vi "Get_Folders_Client.vi"(0 "Relative Path":path) -> (1 "Folder Names":string[](array[string]), 2 "error out":errorcluster)   [LabVIEW 2013]
uses:
  Anemometry/Anemometry Sub Vis/Globals/Preference_global.vi
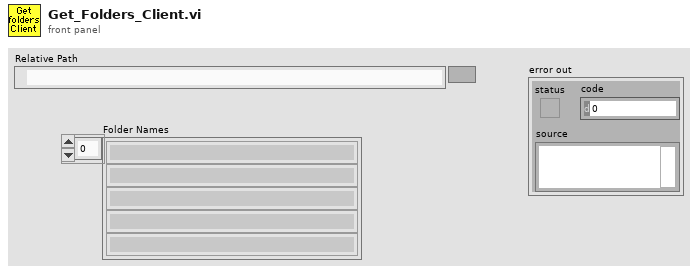
[diagram p1: front panel]
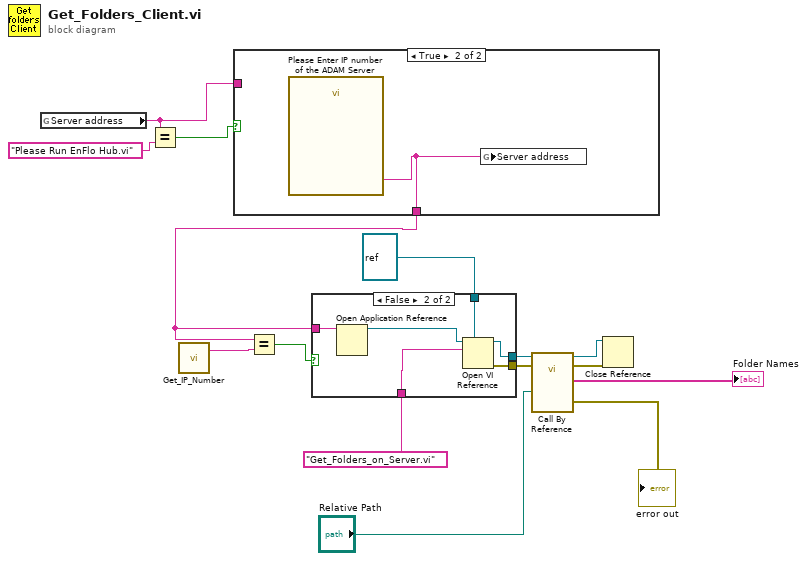
[diagram p0: block diagram]
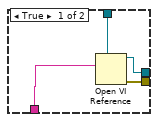
[diagram p3: hidden frame]
diagram:
  n1 = global read "Preference_global.vi" "Server address"() -> (w1:string)
  n2 = Equal?(x=w1, y="Please Run EnFlo Hub.vi" ("Server address")) -> (x = y?=w3:bool)
  n3 = call "Get_IP_Number.vi"() -> ("IP Number"=w9:string)  [unwired: 1 out]
  n4 = case shown="True" w3 {
    tunnel: [w16 w17] -> w2
    tunnel: w1 -> [w16 _]
    frame False {
    }
    frame True {
      n5 = call "Please Enter IP number of the ADAM Server"() -> ("Server IP Number"=w17:string)  [unwired: 17 in, 2 out]
      n6 = global write "Preference_global.vi" "Server address"(w17) -> ()
    }
  }
  n7 = Equal?(x=w2, y=w9) -> (x = y?=w8:bool)
  n8 = case shown="False" w8 {
    tunnel: [w21 w27] -> w10
    tunnel: [w20 w26] -> w11
    tunnel: "Get_Folders_on_Server.vi" -> [w19 w25]
    tunnel: refnum<vi> refnum ("Scout Server") -> [w18 w24]
    tunnel: w2 -> [_ w23]
    frame True {
      n9 = Open VI Reference(type specifier VI Refnum (for type only)=w18, vi path=w19) -> (vi reference=w21:refnum<vi>, error out=w20:errorcluster)  [unwired: 2 in, 2 out]
    }
    frame False {
      n10 = Open Application Reference(11:w23) -> (3:w22:refnum<vi>)  [unwired: 2 in, 2 out]
      n11 = Open VI Reference(type specifier VI Refnum (for type only)=w24, application reference (local)=w22, vi path=w25) -> (vi reference=w27:refnum<vi>, error out=w26:errorcluster)  [unwired: 1 in, 2 out]
    }
  }
  n12 = call-by-ref "?"(reference=w10, error in=w11, "Relative Path"="Relative Path") -> (reference out=w12:refnum<vi>, error out=w15:errorcluster, "Folder Names"=→"Folder Names":string[], "error out"=→"error out":errorcluster)  [unwired: 1 in]
  n13 = Close Reference(reference=w12, error in (no error)=w15) -> ()  [unwired: 1 out]
